vi "Untitled 1 (SubVI).vi"(9 "X":dbl, 10 "Y":dbl) -> (1 "Roll":dbl, 2 "Hover":bool, 3 "Pitch":dbl)   [LabVIEW 2014]
uses:
  Global.vi
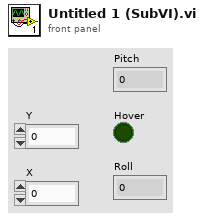
[diagram p1: front panel]
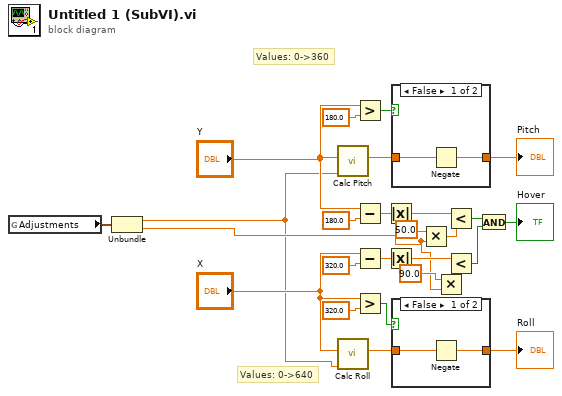
[diagram p0: block diagram]
diagram:
  # "Values: 0->640"
  # "Values: 0->360"
  n1 = global read "Global.vi" "Adjustments"() -> (w3:cluster{"Sensitivity":dbl, "Null Zone":dbl})
  n2 = Unbundle(w3) -> ("Sensitivity"=w1:dbl, "Null Zone"=w2:dbl)
  n3 = call "Calc Pitch.vi"("y"=w1, "Position"="Y") -> ("Pitch"=w21:dbl)  [unwired: 9 in]
  n4 = call "Calc Roll.vi"("y"=w1, "Position"="X") -> ("Roll"=w22:dbl)  [unwired: 9 in]
  n5 = Greater?(x="Y", y=180.0) -> (0:w18:bool)
  n6 = Subtract(x="Y", y=180.0) -> (x-y=w11:dbl)
  n7 = Subtract(x="X", y=320.0) -> (x-y=w23:dbl)
  n8 = Greater?(x="X", y=320.0) -> (0:w20:bool)
  n9 = Absolute Value(x=w11) -> (abs(x)=w13:dbl)
  n10 = Absolute Value(x=w23) -> (abs(x)=w25:dbl)
  n11 = case shown="False" w18 {
    tunnel: w21 -> [w28 w29]
    tunnel: [w27 w29] -> w16
    frame False {
      n12 = Negate(x=w28) -> (-x=w27:dbl)
    }
    frame True {
    }
  }
  "Pitch" <- w16
  n13 = case shown="False" w20 {
    tunnel: w22 -> [w31 w32]
    tunnel: [w30 w32] -> w15
    frame False {
      n14 = Negate(x=w31) -> (-x=w30:dbl)
    }
    frame True {
    }
  }
  "Roll" <- w15
  n15 = Multiply(x=50.0 ("y"), y=w2) -> (x*y=w5:dbl)
  n16 = Multiply(x=90.0 ("y"), y=w2) -> (x*y=w4:dbl)
  n17 = Less?(x=w13, y=w5) -> (x < y?=w9:bool)
  n18 = Less?(x=w25, y=w4) -> (x < y?=w8:bool)
  n19 = And(x=w9, y=w8) -> (x .and. y?=→"Hover":bool)
